vi "basic-lifetime-test.vi"(8 "error in (no error)":errorcluster) -> (0 "error out":errorcluster)   [LabVIEW 2013]
uses:
  src/SMO/SMO.lvclass
  src/SMO/Typedefs/SMOState --Enum.ctl
  <vilib>/addons/_JKI Toolkits/Caraya/classes/Test/Test.lvclass
  <vilib>/addons/_JKI Toolkits/Caraya/classes/Assert/Assert.lvclass
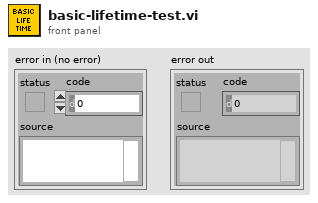
[diagram p1: front panel]
types:
  T1 = typedef "SMO.lvclass/SMOState --Enum.ctl" = enum16{"unknown", "Created", "Started", "Stopped"}
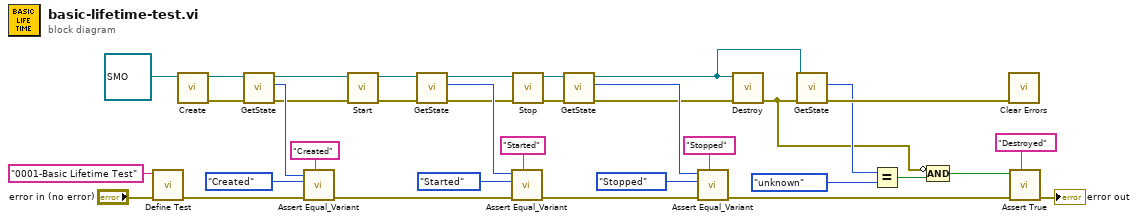
[diagram p0: block diagram]
diagram:
  n1 = call <vilib>:"Define Test.vi"("error in (no error)"="error in (no error)", "Label (VI Title)"="0001-Basic Lifetime Test") -> ("error out"=w31:errorcluster)  [unwired: 9 in]
  n2 = call "Create.vi"("SMO"=refnum<class "SMO.lvclass"> refnum ("SMO.lvclass")) -> ("error out"=w32:errorcluster, "SMO out"=w35:refnum<class "SMO.lvclass">)  [unwired: 8 in, 1 out]
  n3 = call "GetState.vi"("error in (no error)"=w32, "SMO"=w35) -> ("error out"=w27:errorcluster, "SMO State"=w30:T1, "SMO out"=w34:refnum<class "SMO.lvclass">)  [unwired: 7 in]
  n4 = call <vilib>:"Assert Equal_Variant.vi"("Label"="Created" ("Label (VI Title)"), "error in (no error)"=w31, "Y"=SMOState_--Enum."Created" ("SMO State"), "X"=w30) -> ("error out"=w23:errorcluster)  [unwired: 7 in]
  n5 = call "Start.vi"("error in (no error)"=w27, "SMO"=w34) -> ("error out"=w25:errorcluster, "SMO out"=w26:refnum<class "SMO.lvclass">)  [unwired: 8 in]
  n6 = call "GetState.vi"("error in (no error)"=w25, "SMO"=w26) -> ("error out"=w19:errorcluster, "SMO State"=w21:T1, "SMO out"=w20:refnum<class "SMO.lvclass">)  [unwired: 7 in]
  n7 = call <vilib>:"Assert Equal_Variant.vi"("Label"="Started" ("Label (VI Title)"), "error in (no error)"=w23, "Y"=SMOState_--Enum."Started" ("SMO State"), "X"=w21) -> ("error out"=w13:errorcluster)  [unwired: 7 in]
  n8 = call "Stop.vi"("error in (no error)"=w19, "SMO"=w20) -> ("error out"=w16:errorcluster, "SMO out"=w15:refnum<class "SMO.lvclass">)  [unwired: 8 in]
  n9 = call "GetState.vi"("error in (no error)"=w16, "SMO"=w15) -> ("error out"=w12:errorcluster, "SMO State"=w14:T1, "SMO out"=w11:refnum<class "SMO.lvclass">)  [unwired: 7 in]
  n10 = call <vilib>:"Assert Equal_Variant.vi"("Label"="Stopped" ("Label (VI Title)"), "error in (no error)"=w13, "Y"=SMOState_--Enum."Stopped" ("SMO State"), "X"=w14) -> ("error out"=w4:errorcluster)  [unwired: 7 in]
  n11 = call "Destroy.vi"("error in (no error)"=w12, "SMO"=w11) -> ("error out"=w5:errorcluster)  [unwired: 9 in]
  n12 = call "GetState.vi"("error in (no error)"=w5, "SMO"=w11) -> ("error out"=w9:errorcluster, "SMO State"=w7:T1)  [unwired: 7 in, 1 out]
  n13 = Equal?(x=w7, y=SMOState_--Enum."unknown" ("SMO State")) -> (x = y?=w6:bool)
  n14 = Compound Arithmetic op=AND(invert w5, w6) -> (w1:bool)
  n15 = call <vilib>:"Clear Errors.vi"("error in (no error)"=w9) -> ()  [unwired: 6 in, 1 out]
  n16 = call <vilib>:"Assert True.vi"("Label"="Destroyed" ("Label (VI Title)"), "error in (no error)"=w4, "True?"=w1) -> ("error out"=→"error out":errorcluster)  [unwired: 8 in]
